vi "Create Linearity Results Summary Table.vi"(8 "error in (no error)":errorcluster, 11 "Linearity Results":T1[](array[typedef]) {"Linearity Percent FS" format="%#_3g"}) -> (0 "error out":errorcluster, 3 "Linearity Table":string[][](array[string]))   [LabVIEW 2026, in "Analysis.lvlib"]
uses:
  Analysis.lvlib
  Linearity Result.ctl
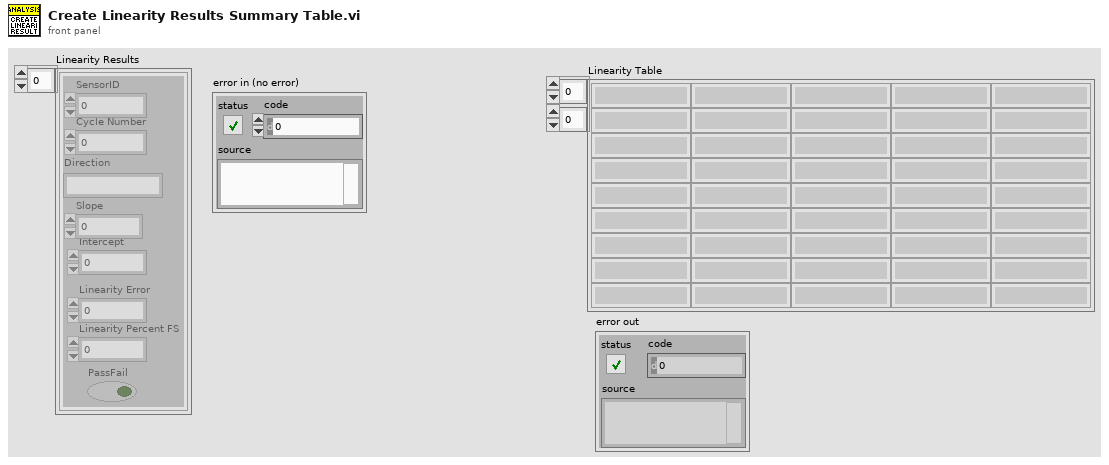
[diagram p1: front panel]
types:
  T1 = typedef "Analysis.lvlib/Linearity Result.ctl" = cluster{"Slope":dbl, "Intercept":dbl, "Cycle Number":i32, "SensorID":i32, "Linearity Error":dbl, "Linearity Percent FS":dbl, "Direction":string, "PassFail":bool}
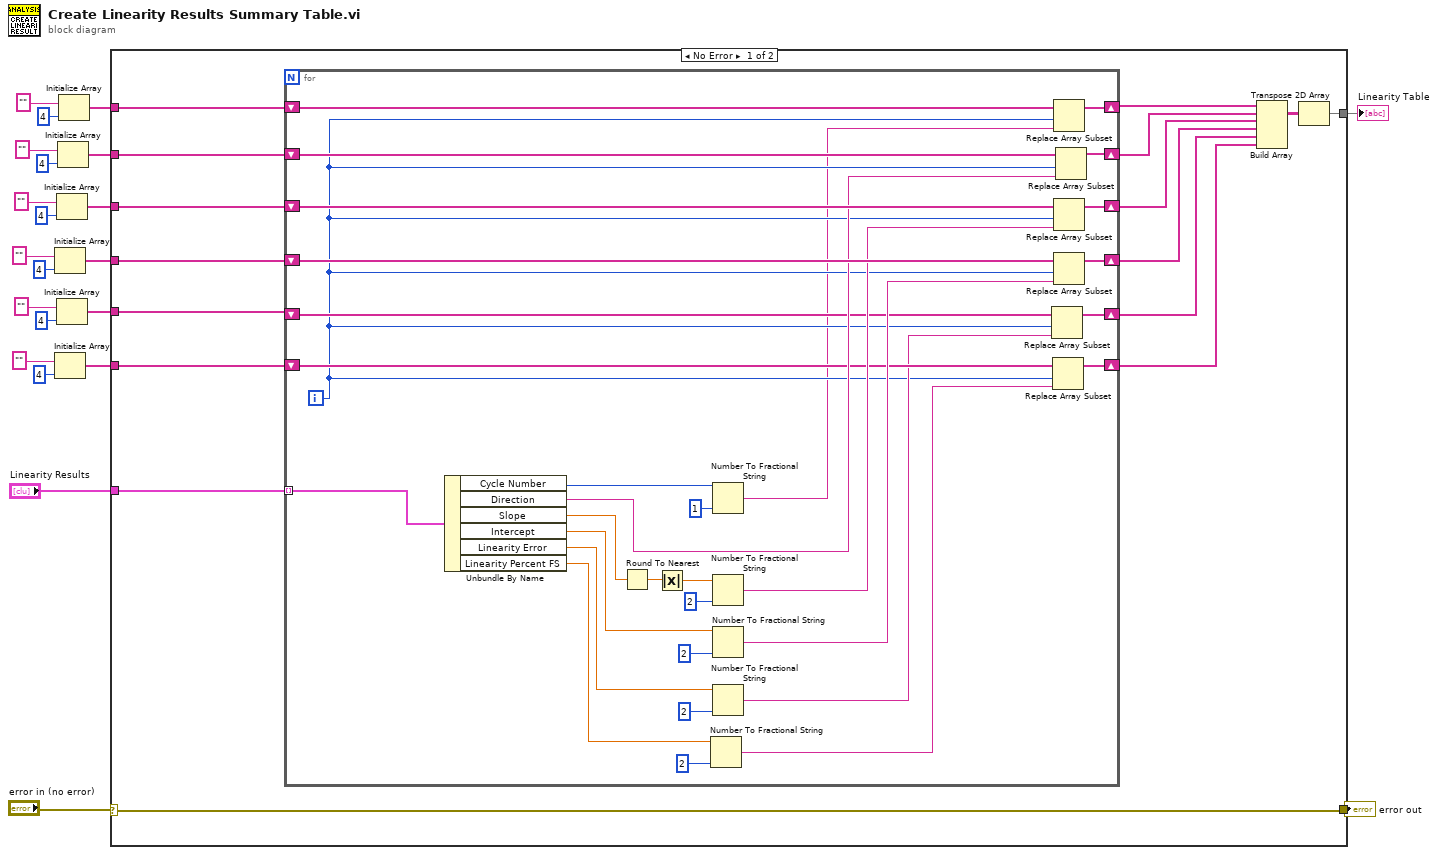
[diagram p0: block diagram]
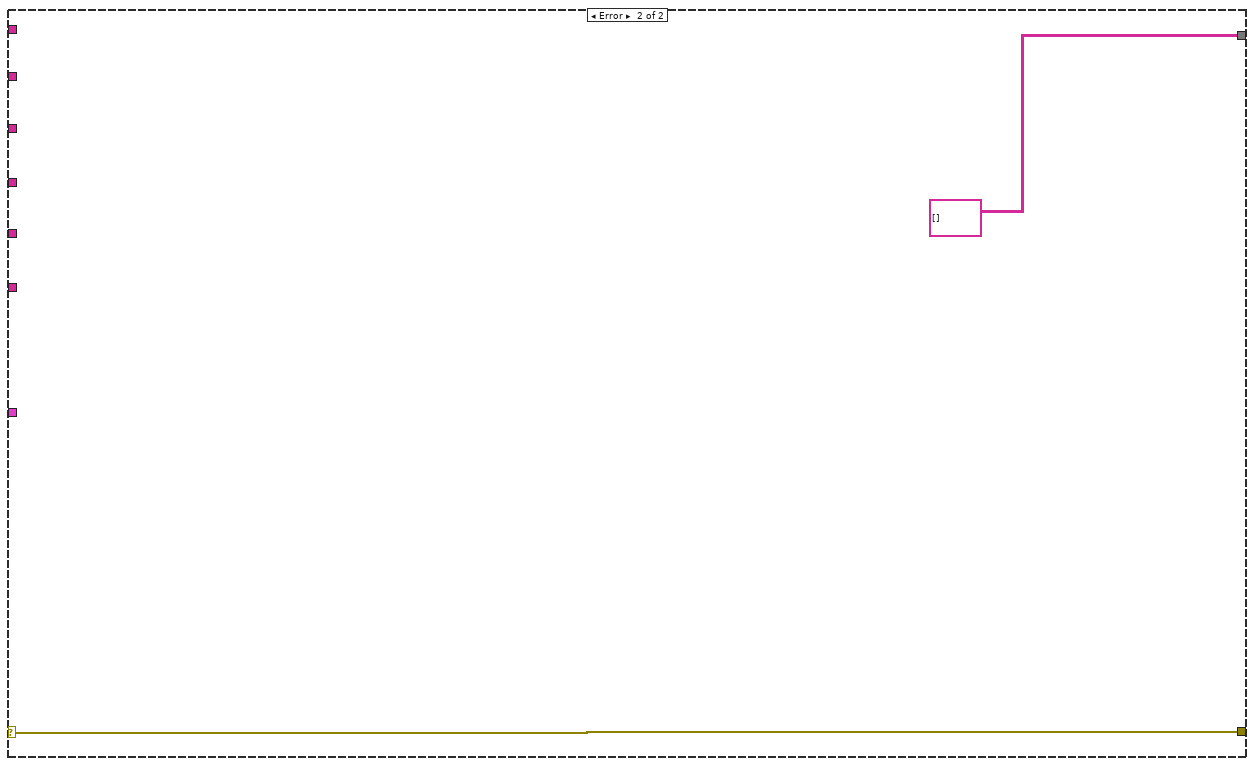
[diagram p2: hidden frame]
diagram:
  n1 = Initialize Array("" ("element"), 4 ("dimension size")) -> (w8:string[])
  n2 = Initialize Array("" ("element"), 4 ("dimension size")) -> (w2:string[])
  n3 = Initialize Array("" ("element"), 4 ("dimension size")) -> (w11:string[])
  n4 = Initialize Array("" ("element"), 4 ("dimension size")) -> (w3:string[])
  n5 = Initialize Array("" ("element"), 4 ("dimension size")) -> (w17:string[])
  n6 = Initialize Array("" ("element"), 4 ("dimension size")) -> (w20:string[])
  n7 = case shown="No Error" "error in (no error)" {
    selector: "error in (no error)" -> [w32 w72]
    tunnel: w20 -> [w38 _]
    tunnel: w17 -> [w37 _]
    tunnel: "Linearity Results" -> [w23 _]
    tunnel: [w33 string[][] []] -> w16
    tunnel: [w32 w72] -> w14
    tunnel: w11 -> [w31 _]
    tunnel: w8 -> [w29 _]
    tunnel: w3 -> [w27 _]
    tunnel: w2 -> [w25 _]
    frame No Error {
      n8 = for {
        shift-right: [w69] -> w36
        shift-left: w38 -> [w70]
        shift-right: [w67] -> w35
        shift-left: w37 -> [w68]
        shift-right: [w65] -> w30
        shift-left: w31 -> [w66]
        shift-right: [w63] -> w28
        shift-left: w29 -> [w64]
        tunnel: w23 -> [w39] mode=indexing
        shift-right: [w46] -> w26
        shift-left: w27 -> [w47]
        shift-right: [w44] -> w24
        shift-left: w25 -> [w45]
        i -> [w41]
        n9 = Unbundle By Name(w39) -> ("Cycle Number"=w57:i32, "Direction"=w56:string, "Slope"=w55:dbl, "Intercept"=w52:dbl, "Linearity Error"=w50:dbl, "Linearity Percent FS"=w48:dbl)
        n10 = Round To Nearest(number=w55) -> (nearest integer value=w54:dbl)
        n11 = Absolute Value(x=w54) -> (abs(x)=w53:dbl)
        n12 = Number To Fractional String(number=w48, precision (6)=i16 2) -> (F-format string=w42:string)  [unwired: 2 in]
        n13 = Number To Fractional String(number=w57, precision (6)=i16 1) -> (F-format string=w40:string)  [unwired: 2 in]
        n14 = Number To Fractional String(number=w53, precision (6)=i16 2) -> (F-format string=w62:string)  [unwired: 2 in]
        n15 = Number To Fractional String(number=w52, precision (6)=i16 2) -> (F-format string=w61:string)  [unwired: 2 in]
        n16 = Number To Fractional String(number=w50, precision (6)=i16 2) -> (F-format string=w43:string)  [unwired: 2 in]
        n17 = Replace Array Subset(array=w47, new element=w43, index=w41) -> (w46:string[])
        n18 = Replace Array Subset(array=w45, new element=w42, index=w41) -> (w44:string[])
        n19 = Replace Array Subset(array=w70, new element=w40, index=w41) -> (w69:string[])
        n20 = Replace Array Subset(array=w66, new element=w62, index=w41) -> (w65:string[])
        n21 = Replace Array Subset(array=w64, new element=w61, index=w41) -> (w63:string[])
        n22 = Replace Array Subset(array=w68, new element=w56, index=w41) -> (w67:string[])
      }
      n23 = Build Array(w36, w35, w30, w28, w26, w24) -> (w34:string[][])
      n24 = Transpose 2D Array(2D array=w34) -> (transposed array=w33:string[][])
    }
    frame Error {
    }
  }
  "Linearity Table" <- w16
  "error out" <- w14
